vi "LoadCrvEdPanel.vi"(4 "EditorProgQEvent":refnum<user-event>, 6 "EditorProgQ":refnum<queue>, 8 "error in (no error)":errorcluster caption="entrée d'erreur (pas d'erreur)", 11 "RemPanRef":refnum<vi>) -> (0 "sortie d'erreur":errorcluster, 2 "ViNameOut":string[](array[string]), 3 "PanelViRefOut":refnum<vi>[](array[refnum]))   [LabVIEW 2019]
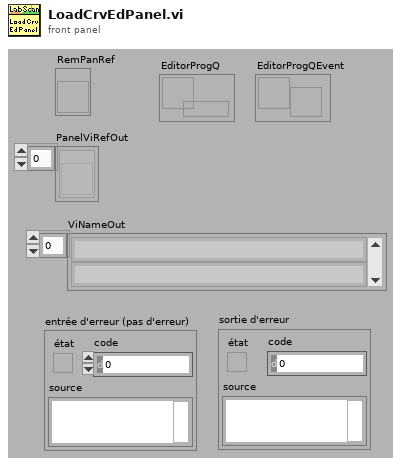
[diagram p1: front panel]
types:
  T1 = enum16{"Répertoire du VI actuel", "Répertoire du parent 1", "Répertoire du parent 2", "Répertoire du parent 3"}
  T2 = typedef "LVPointTypeDef.ctl" = cluster{"Horizontal":i16, "Vertical":i16}
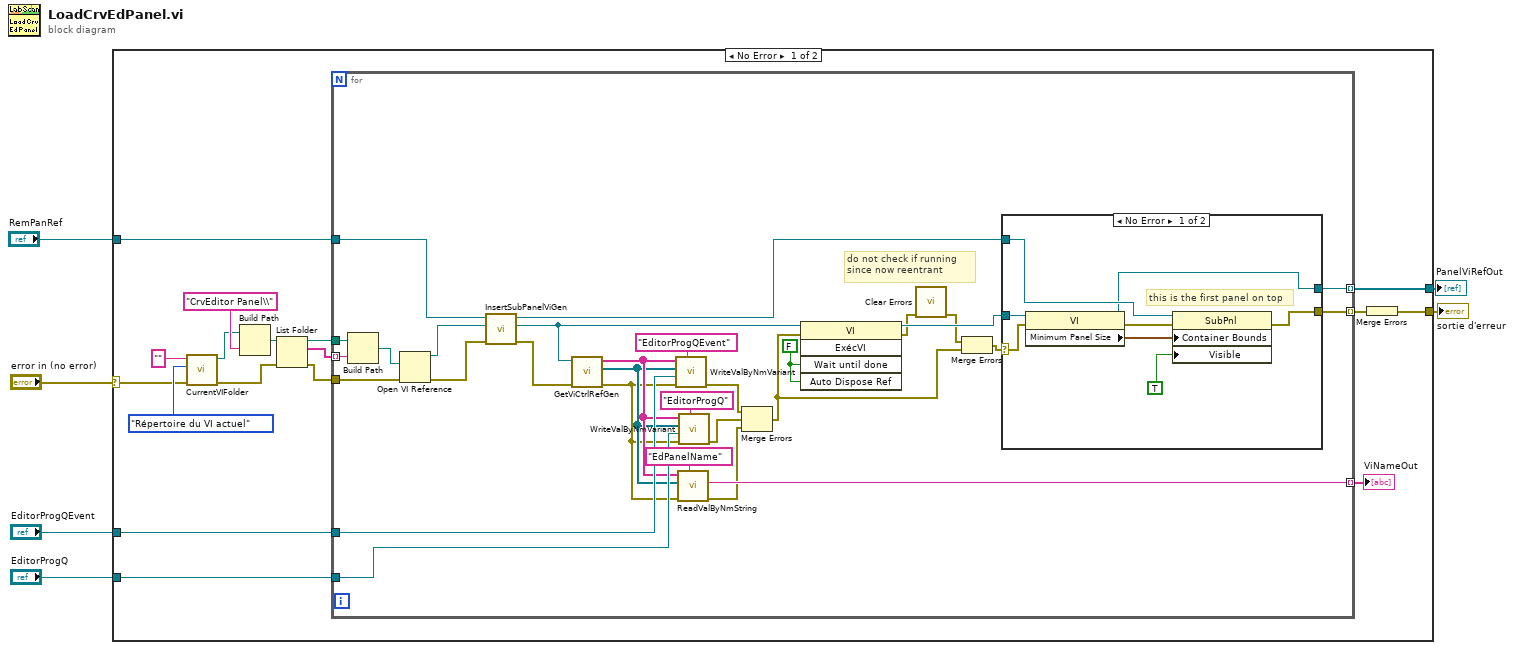
[diagram p0: block diagram]
diagram:
  n1 = case shown="No Error" "error in (no error)" {
    selector: "error in (no error)" -> [w10 w64]
    tunnel: [w23 w64] -> w5
    tunnel: "EditorProgQEvent" -> [w22 _]
    tunnel: "EditorProgQ" -> [w21 _]
    tunnel: "RemPanRef" -> [w19 _]
    tunnel: [w8 _] -> w1
    frame No Error {
      n2 = call <userlib>:"CurrentVIFolder.vi"("error in (no error)"=w10, "Source"=T1."Répertoire du VI actuel", "NomFichier"="") -> ("error out"=w16:errorcluster, "Chemin"=w13:path)  [unwired: 6 in, 1 out]
      n3 = Build Path(base path=w13, name or relative path="CrvEditor Panel\\" ("nom ou chemin relatif")) -> (appended path=w15:path)
      n4 = List Folder(path=w15, error in=w16) -> (path out=w12:path, filenames=w11:string[], error out=w9:errorcluster)  [unwired: 2 in, 1 out]
      n5 = for {
        tunnel: w9 -> [w28]
        tunnel: [w51] -> w20 mode=indexing
        tunnel: w22 -> [w43]
        tunnel: w21 -> [w42]
        tunnel: w19 -> [w30]
        tunnel: w12 -> [w50]
        tunnel: w11 -> [w49] mode=indexing
        tunnel: [w47] -> w8 mode=indexing
        tunnel: [w35] -> w7 mode=indexing
        w52 = FALSE ("Attendre la fin")
        # "do not check if running \nsince now reentrant"
        n6 = Build Path(base path=w50, name or relative path=w49) -> (appended path=w48:path)
        n7 = Open VI Reference(vi path=w48, error in (no error)=w28) -> (vi reference=w26:refnum<vi>, error out=w27:errorcluster)  [unwired: 4 in]
        n8 = call <userlib>:"InsertSubPanelViGen.vi"("error in (no error)"=w27, "RemVIRef"=w26, "RemPanRef"=w30) -> ("sortie d'erreur"=w24:errorcluster, "RemVIRefOut"=w25:refnum<vi>, "RemPanRefOut"=w29:refnum<vi>)  [unwired: 6 in]
        n9 = call <userlib>:"GetViCtrlRefGen.vi"("ErrorIn(No Error)"=w24, "VIRef"=w25) -> ("sortie d'erreur"=w36:errorcluster, "ControlsRefs"=w37:refnum<vi>[], "ControlsNames"=w38:string[])  [unwired: 7 in]
        n10 = call <userlib>:"WriteValByNmVariant.vi"("Ctrl Name"="EditorProgQEvent" ("élément"), "error in"=w36, "Valeur"=w43, "CtrlRef"=w37, "ControlsNames"=w38) -> ("error out"=w33:errorcluster)  [unwired: 5 in, 1 out]
        n11 = call <userlib>:"ReadValByNmString.vi"("Ctrl Name"="EdPanelName" ("élément"), "error in"=w36, "CtrlRef"=w37, "ControlsNames"=w38) -> ("error out"=w31:errorcluster, "Valeur"=w35:string)  [unwired: 5 in, 1 out]
        n12 = call <userlib>:"WriteValByNmVariant.vi"("Ctrl Name"="EditorProgQ" ("élément"), "error in"=w36, "Valeur"=w42, "CtrlRef"=w37, "ControlsNames"=w38) -> ("error out"=w32:errorcluster)  [unwired: 5 in, 1 out]
        n13 = Merge Errors(w33, w32, w31) -> (w34:errorcluster)
        n14 = invoke class="VI" method="ExécVI"(reference=w25, error in=w34, "Wait until done"=w52, "Auto Dispose Ref"=w52) -> (reference out=w53:refnum<vi>, error out=w45:errorcluster)  [unwired: 1 in, 3 out]
        n15 = call <vilib>:"Clear Errors.vi"("error in (no error)"=w45) -> ("error out"=w44:errorcluster)  [unwired: 5 in, 1 out]
        n16 = Merge Errors(w44, w34) -> (w46:errorcluster)
        n17 = case shown="No Error" w46 {
          selector: w46 -> [w58 w63]
          tunnel: [w56 w63] -> w51
          tunnel: w29 -> [w59 _]
          tunnel: w53 -> [w57 w62]
          tunnel: [w54 w62] -> w47
          frame No Error {
            # "this is the first panel on top"
            n18 = property class="VI"(reference=w57, error in=w58) -> (reference out=w54:refnum<vi>, error out=w60:errorcluster, "Minimum Panel Size"=w61:T2)
            n19 = property class="SubPnl"(reference=w59, error in=w60, "Container Bounds"=w61, "Visible"=TRUE) -> (error out=w56:errorcluster)  [unwired: 1 out]
          }
          frame Error {
          }
        }
      }
      "ViNameOut" <- w7
      n20 = Merge Errors(w20) -> (w23:errorcluster)
    }
    frame Error {
    }
  }
  "sortie d'erreur" <- w5
  "PanelViRefOut" <- w1
